vi "Set Receive Channel [RXN].vi"(7 "Micropulse # In":i32, 8 "error in (no error)":errorcluster, 9 "Probe Number":i32=-1 caption="Probe Number [def: Not assigned]", 10 "Channel Number":u32, 11 "Test Number":u32) -> (0 "error out":errorcluster, 5 "Micropulse # Out":i32)   [LabVIEW 2026, in "MicroPulse_Driver.lvlib"]
doc: "Selects the receiver probe connection for a given test number (Tn).\n\nParameters:\n<Tn>:Test number. An integer value from 0 to the maximum number of tests (default maximum is 1279 tests).\nTn = 0 for all tests.\n\n<Channel>:Integer in the range of 1 to the maximum number of focal laws (default 1024). When the <Tn> is 256 or greater, this parameter refers to a phased array focal law and not an actual MicroPulse channel.\n\n[Vpn]:Optional probe number.\nIf channel is set to 0 then this integer value from 1 to 16 specifies a virtual probe consisting of conventional channels.\n\nExample:\nRXN 7 4 :Assigns pulser/receiver channel 4 as receiver for Test Number 7.\nRXN 256 1 :Assigns receive phased array focal law 1 to test 256."
uses:
  MicroPulse_Driver.lvlib
  Private/MP-Registry Action-Enum.ctl
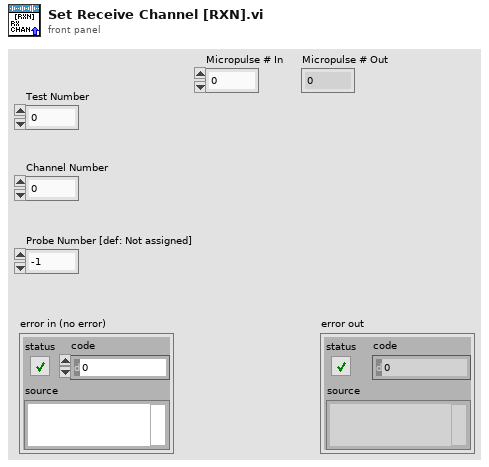
[diagram p1: front panel]
types:
  T1 = typedef "MicroPulse_Driver.lvlib/MP-Registry Action-Enum.ctl" = enum16{"Read", "Add Test", "Add Command", "Add Gate Command", "Add Encoder Command", "Clear Command  List", "Set Registry", "Set System Details", "Set DOF", "Set Velocity", "Disable Asynch Reads", "Enable Asynch Reads", "Add Connection", "Disconnect", "Shutdown"}
  T2 = typedef "MicroPulse_Driver.lvlib/TCP config.ctl" = cluster{"Connection ID":refnum<k5>, "IP address":string, "host port":u16, "OC timeout":i32, "Read timeout":i32, "Write timeout":i32}
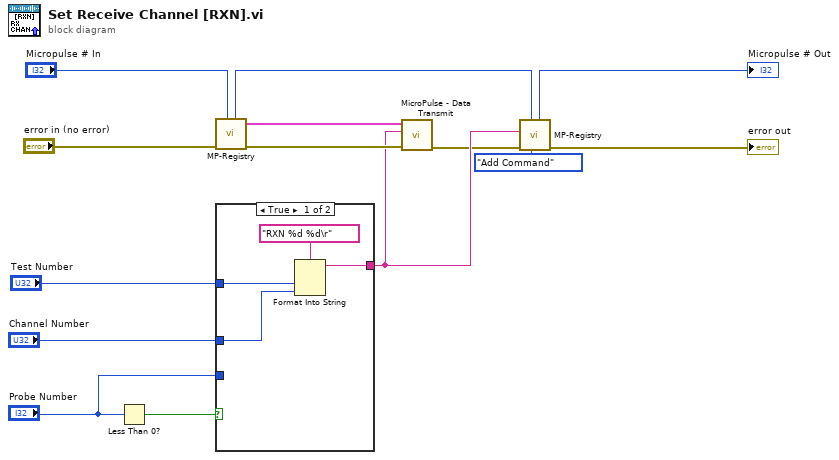
[diagram p0: block diagram]
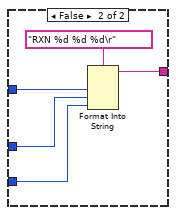
[diagram p2: hidden frame]
diagram:
  n1 = Less Than 0?(x="Probe Number") -> (x < 0?=w9:bool)
  n2 = call "MP-Registry.vi"("Micropulse # In"="Micropulse # In", "error in (no error)"="error in (no error)") -> ("error out"=w12:errorcluster, "TCP config"=w11:T2, "Micropulse # Out"=w2:i32)  [unwired: 6 in, 1 out]
  n3 = case shown="True" w9 {
    tunnel: "Test Number" -> [w17 w22]
    tunnel: "Channel Number" -> [w16 w21]
    tunnel: "Probe Number" -> [_ w20]
    tunnel: [w15 w19] -> w6
    frame True {
      n4 = Format Into String(format string="RXN %d %d\r", w17, w16) -> (resulting string=w15:string)  [unwired: 2 in, 1 out]
    }
    frame False {
      n5 = Format Into String(format string="RXN %d %d %d\r", w22, w21, w20) -> (resulting string=w19:string)  [unwired: 2 in, 1 out]
    }
  }
  n6 = call "MicroPulse - Data Transmit.vi"("error in (no error)"=w12, "data"=w6, "TCP config"=w11) -> ("error out"=w4:errorcluster)  [unwired: 6 in, 2 out]
  n7 = call "MP-Registry.vi"("Action"=MP-Registry_Action-Enum."Add Command", "Micropulse # In"=w2, "error in (no error)"=w4, "Data in"=w6) -> ("error out"=→"error out":errorcluster, "Micropulse # Out"=→"Micropulse # Out":i32)  [unwired: 4 in, 2 out]
